vi "Standard Bus LabView Example.vi"() -> ()   [LabVIEW 2018]
uses:
  Example Cntl.ctl
  C:/RageATE/Instruments/Ess Temp Plate/LabView Driver/Public/Watbus.dll
  Watbus.dll
panel:
  in  "7. Temperature Units":u8(ring) items=["Degrees F", "Degrees C"]
  in  "Interface":i32(ring)=1 caption="1. Interface" items=["USB", "Serial", "Ethernet"]
  in  "4. ZONE":i32=1 min=1 max=17
  in  "6. Instance ID":i32=1 min=0 max=255 step=1
  out "Error out":errorcluster
  out "Connected?":bool
  in  "Initalize":bool
  in  "Read":bool
  in  "Write":bool
  in  "Close":bool
  in  "Exit":bool
  in  "Write Value":string
  in  "EZ-ZONE Port":refnum<visa-resource-name>="COM1" caption="2. EZ-ZONE Port"
  in  "3. Device Type":i32(ring) items=["Controller", "RUI", "PC", "CommsCard"]
  in  "5. Parameter ID":i32=4001 min=1001 max=100000 step=1
  out "Value Out":string
  # "Standard Bus  Example VI"
  # "1.   Interface :\n      0- USB (not used)\n      1- Serial (RS-232 or USB to EIA-485 converter)\n      2 -Ethernet (D4T & F4T only)\n2.   Watlow Port :\n       USB - Enter controller Serial Number\n       Serial - Select or enter available Serial Port\n                    Example: COM1, COM2, COM3, ....\n       Ethernet - Enter IP Address\n                         Example: 192.168.0.222 \n3.    Device Type :\n       Controller - Any EZ-ZONE controller\n       RUI - Any EZ-ZONE Remote User Interface\n       PC - (not used)\n       Commscard - (not used)\n4.   ZONE :\n      Address (1 to 17) of controller. Use 1 for Ethernet device.\n5.   Parameter ID :\n      Enter Parameter ID to read/write. Refer to  user's guide or\n      Excel Spreadsheet for Parameter ID and Instance ID.\n6.   Instance number :\n      Instance number refers to occurrence of the parameter.\n      Example: Analog Input 1 = Instance 1 of the input.\n                       Analog Input 2 = Instance 2 of the input.\n                       Alarm 1 = Instance 1  of the alarm.\n                       Alarm 2 = Instance 2 of the alarm.\n7. Temperatue Units :\n      Choose display units applied to temperature related parameter values.\n8.   Initialize :\n      Click to open port first time. Connected? turns green.\n9.   Read :\n      Click to read the parameter specified.\n      Value Out contains result. Temperature in °F if applicable.\n10.   Write :\n       Enter Write Value, then click when changing a parameter.\n       Temperature in °F or °C if applicable.\n11.  Close :\n        Select to close the communications connection.\n12   Exit :\n       Select to exit the application.\nStatus & Code\n        Success = 0, green check mark\n        Failure = non-zero, red X\nError Out : verbose read/write request results"
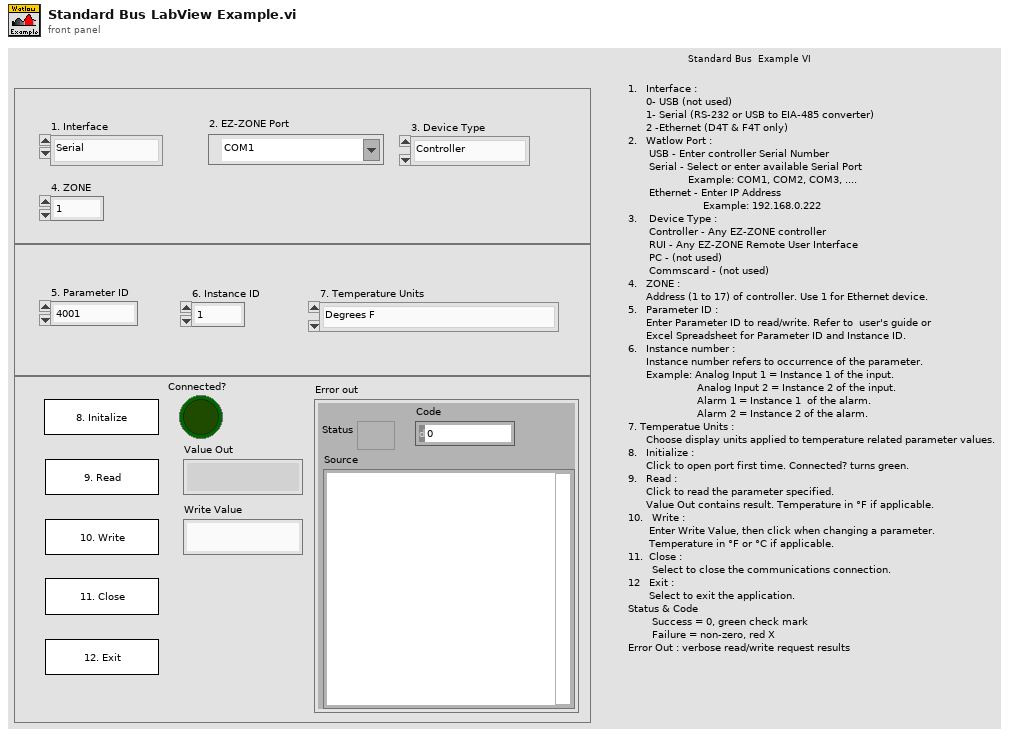
[diagram p1: front panel]
types:
  T1 = typedef "Example Cntl.ctl" = enum16{"Initialize", "Read", "Write", "Close", "Exit"}
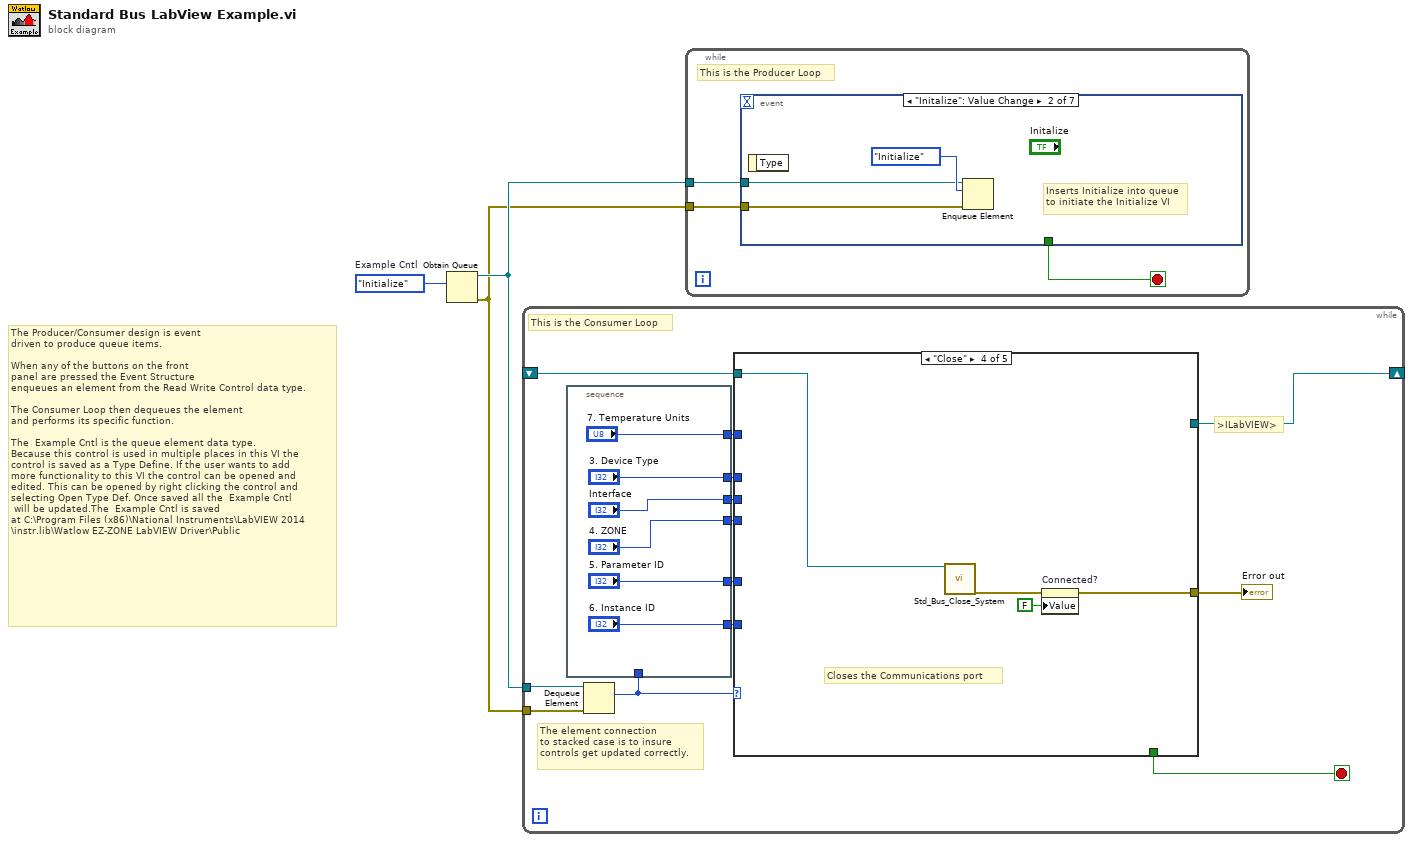
[diagram p0: block diagram]
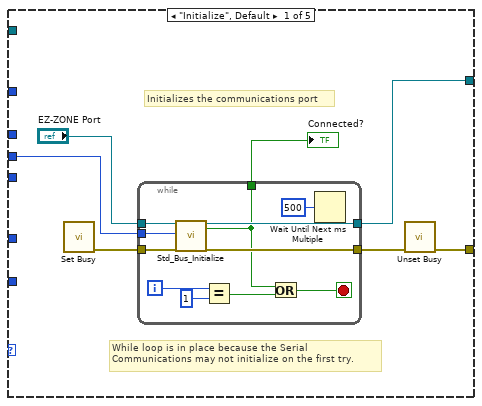
[diagram p2: hidden frame]
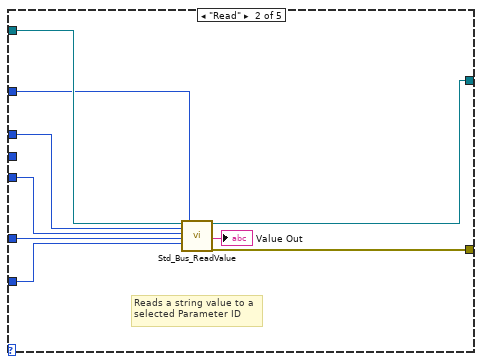
[diagram p3: hidden frame]
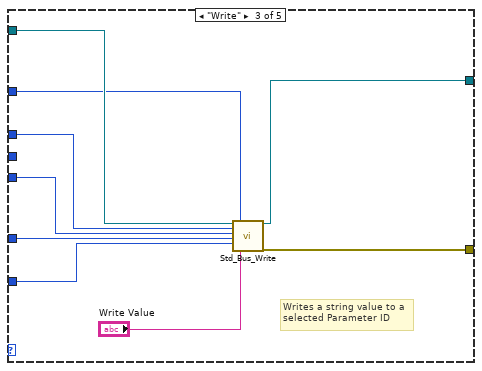
[diagram p4: hidden frame]
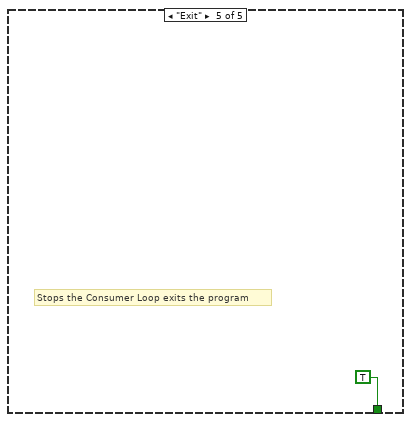
[diagram p5: hidden frame]
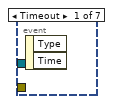
[diagram p6: hidden frame]
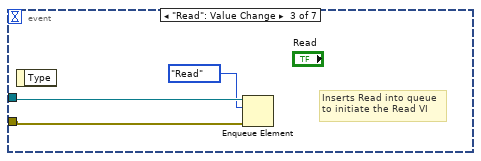
[diagram p7: hidden frame]
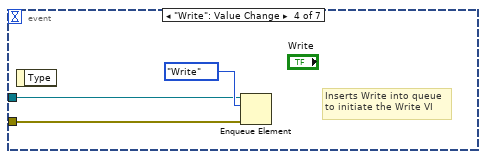
[diagram p8: hidden frame]
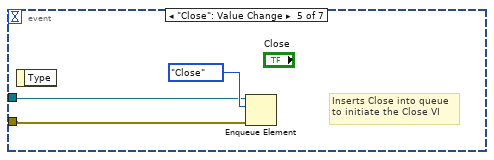
[diagram p9: hidden frame]
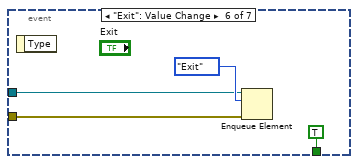
[diagram p10: hidden frame]
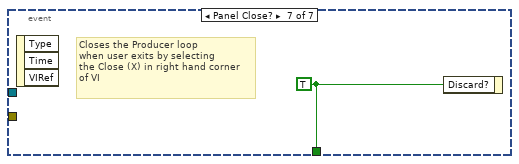
[diagram p11: hidden frame]
diagram:
  w3 = Example_Cntl."Initialize"  # Example Cntl
  # "The Producer/Consumer design is event\ndriven to produce queue items.\n\nWhen any of the buttons on the front\npanel are pressed the Event Structure \nenqueues an element from the Read Write Control data type.\n\nThe Consumer Loop then dequeues the element\nand performs its specific function.\n\nThe  Example Cntl is the queue element data type.\nBecause this control is used in multiple places in this VI the\ncontrol is saved as a Type Define. If the user wants to add\nmore functionality to this VI the control can be opened and\nedited. This can be opened by right clicking the control and\nselecting Open Type Def. Once saved all the  Example Cntl \n will be updated.The  Example Cntl is saved \nat C:\\Program Files (x86)\\National Instruments\\LabVIEW 2014\n\\instr.lib\\Watlow EZ-ZONE LabVIEW Driver\\Public"
  n1 = Obtain Queue(element data type=w3) -> (queue out=w2:refnum<queue>, error out=w1:errorcluster)  [unwired: 4 in, 1 out]
  n2 = while {
    tunnel: w1 -> [w16]
    tunnel: w2 -> [w15]
    shift-right: [w12] -> _
    shift-left: _ -> [w11]
    stop <- w8 stop-if-true
    # ">ILabVIEW>"
    # "The element connection\nto stacked case is to insure\ncontrols get updated correctly."
    # "This is the Consumer Loop"
    n3 = Dequeue Element(queue=w15, error in (no error)=w16) -> (element=w14:T1)  [unwired: 4 out]
    n4 = stacked-sequence {
      tunnel: w14 -> [_]
      tunnel: ["Interface"] -> w13
      tunnel: ["6. Instance ID"] -> w10
      tunnel: ["4. ZONE"] -> w7
      tunnel: ["3. Device Type"] -> w6
      tunnel: ["5. Parameter ID"] -> w5
      tunnel: ["7. Temperature Units"] -> w4
      frame #0 {
      }
    }
    n5 = case shown="\"Close\"" w14 {
      tunnel: w13 -> [w28 _ _ _ _]
      tunnel: [w25 w48 w57 _ _] -> w12
      tunnel: w11 -> [_ w49 w58 w59 _]
      tunnel: w10 -> [_ w42 w52 _ _]
      tunnel: [w29 w47 w55 w60 _] -> w9
      tunnel: [_ _ _ _ TRUE] -> w8
      tunnel: w7 -> [_ w46 w53 _ _]
      tunnel: w6 -> [_ w44 w54 _ _]
      tunnel: w5 -> [_ w45 w51 _ _]
      tunnel: w4 -> [_ w41 w50 _ _]
      frame "Initialize", Default {
        # "While loop is in place because the Serial\nCommunications may not initialize on the first try."
        # "Initializes the communications port"
        n6 = call <vilib>:"Set Busy.vi"() -> ("error out"=w23:errorcluster)  [unwired: 4 in, 7 out]
        n7 = while {
          tunnel: w28 -> [w31]
          tunnel: "EZ-ZONE Port" -> [w30]
          tunnel: [w34] -> w26
          tunnel: [w40] -> w25
          tunnel: w23 -> [w38]
          tunnel: [w39] -> w24
          i -> [w37]
          stop <- w33 stop-if-true
          n8 = call "Std_Bus_Initialize.vi"("Communications Port"=w30, "InterfaceType"=w31, "error in (no error)"=w38) -> ("IsConnected"=w34:bool, "ILabVIEW"=w40:refnum<k24>, "error out"=w39:errorcluster)  [unwired: 14 out]
          n9 = Equal?(x=w37, y=1) -> (x = y?=w35:bool)
          n10 = Or(x=w34, y=w35) -> (x .or. y?=w33:bool)
          n11 = Wait Until Next ms Multiple(millisecond multiple=u32 500) -> ()  [unwired: 1 out]
        }
        "Connected?" <- w26
        n12 = call <vilib>:"Unset Busy.vi"("error in (no error)"=w24) -> ("error out"=w29:errorcluster)  [unwired: 1 in, 9 out]
      }
      frame "Read" {
        # "Reads a string value to a\nselected Parameter ID"
        n13 = call "Std_Bus_ReadValue.vi"("ILabVIEW In"=w49, "DeviceType"=w44, "Zone"=w46, "ParameterID"=w45, "InstanceId"=w42, "TemperatureUnits"=w41) -> ("ILabVIEW Out"=w48:refnum<k24>, "Value Out"=→"Value Out":string, "error out"=w47:errorcluster)  [unwired: 1 in, 10 out]
      }
      frame "Write" {
        # "Writes a string value to a\nselected Parameter ID"
        n14 = call "Std_Bus_Write.vi"("ILabVIEW In"=w58, "deviceType"=w54, "Zone"=w53, "ParameterID"=w51, "InstanceId"=w52, "TemperatureUnits"=w50, "WriteValue"="Write Value") -> ("ILabVIEW Out"=w57:refnum<k24>, "error out"=w55:errorcluster)  [unwired: 1 in, 10 out]
      }
      frame "Close" {
        # "Closes the Communications port"
        n15 = call "Std_Bus_Close_System.vi"("ILabVIEW In"=w59) -> ("error out"=w61:errorcluster)  [unwired: 1 in, 17 out]
        n16 = property on="Connected?" class="Bool (strict)"(error in=w61, "Value"=FALSE ("IsConnected")) -> (error out=w60:errorcluster)  [unwired: 1 in, 1 out]
      }
      frame "Exit" {
        # "Stops the Consumer Loop exits the program"
      }
    }
    "Error out" <- w9
  }
  n17 = while {
    tunnel: w2 -> [w66]
    tunnel: w1 -> [w65]
    stop <- w64 stop-if-true
    # "This is the Producer Loop"
    n18 = event shown="[1] \"Initalize\": Value Change" {
      selector: _ -> [_ _ _ _ _ _ _]
      dyn-events: _ -> [_ _ _ _ _ _ _]
      timeout: _ -> [_ _ _ _ _ _ _]
      tunnel: w66 -> [_ w68 w72 w74 w77 w81 _]
      tunnel: w65 -> [_ w67 w71 w73 w76 w80 _]
      tunnel: [_ _ _ _ _ TRUE ("Discard?") w83] -> w64
      event Timeout {
        n19 = event-data() -> ()  [unwired: 3 out]
      }
      event "Initalize": Value Change {
        # "Inserts Initialize into queue\nto initiate the Initialize VI"
        n20 = event-data() -> ()  [unwired: 2 out]
        n21 = Enqueue Element(queue=w68, element=Example_Cntl."Initialize" ("Enum"), error in (no error)=w67) -> ()  [unwired: 4 out]
      }
      event "Read": Value Change {
        # "Inserts Read into queue\nto initiate the Read VI"
        n22 = event-data() -> ()  [unwired: 2 out]
        n23 = Enqueue Element(queue=w72, element=Example_Cntl."Read" ("Enum"), error in (no error)=w71) -> ()  [unwired: 4 out]
      }
      event "Write": Value Change {
        # "Inserts Write into queue\nto initiate the Write VI"
        n24 = event-data() -> ()  [unwired: 2 out]
        n25 = Enqueue Element(queue=w74, element=Example_Cntl."Write" ("Enum"), error in (no error)=w73) -> ()  [unwired: 4 out]
      }
      event "Close": Value Change {
        # "Inserts Close into queue\nto initiate the Close VI"
        n26 = event-data() -> ()  [unwired: 2 out]
        n27 = Enqueue Element(queue=w77, element=Example_Cntl."Close" ("Enum"), error in (no error)=w76) -> ()  [unwired: 4 out]
      }
      event "Exit": Value Change {
        n28 = event-data() -> ()  [unwired: 2 out]
        n29 = Enqueue Element(queue=w81, element=Example_Cntl."Exit" ("Enum"), error in (no error)=w80) -> ()  [unwired: 4 out]
      }
      event Panel Close? {
        w83 = TRUE ("Discard?")
        # "Closes the Producer loop\nwhen user exits by selecting\nthe Close (X) in right hand corner\nof VI"
        n30 = event-data() -> ()  [unwired: 4 out]
        n31 = event-data("Discard?"=w83) -> ()  [unwired: 1 in, 1 out]
      }
    }
  }
